vi "Configure Sweep Mode.vi"(8 "error in (no error)":errorcluster, 10 "Sweep Mode":enum16{"Continuous", "Single"}(ring), 11 "SA-ESA in":refnum<class "SA-ESA.lvclass">) -> (0 "error out":errorcluster, 3 "SA-ESA out":refnum<class "SA-ESA.lvclass">)   [LabVIEW 2020, in "SA-ESA.lvclass"]
uses:
  SA-ESA.lvclass
  C:/Sandbox/Git_Sandbox/WiSpry Test Framework source code (LV20)/WiSpry Test Framework/Instruments/Instrument.lvclass
  Instrument.lvclass/Instrument.ctl
  Instrument.lvclass
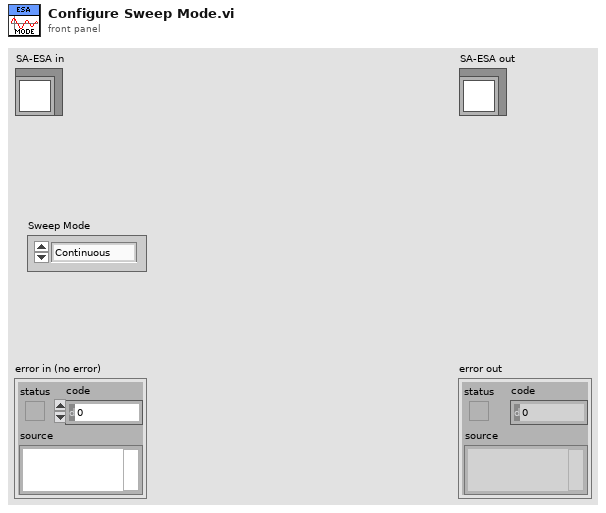
[diagram p1: front panel]
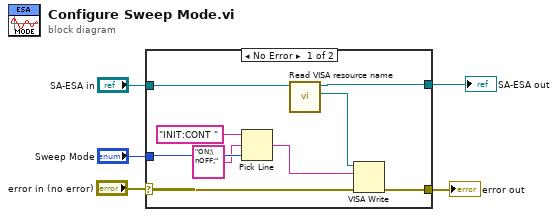
[diagram p0: block diagram]
diagram:
  n1 = case shown="No Error" "error in (no error)" {
    selector: "error in (no error)" -> [w8 w15]
    tunnel: "SA-ESA in" -> [w11 w16]
    tunnel: "Sweep Mode" -> [w14 _]
    tunnel: [w7 w15] -> w2
    tunnel: [w6 w16] -> w1
    frame No Error {
      n2 = Pick Line(string ("")="INIT:CONT ", multi-line string="ON;\nOFF;", line index=w14) -> (output string=w9:string)
      n3 = call "Read VISA resource name.vi"("Instrument in"=w11) -> ("VISA resource name"=w10:refnum<visa-resource-name>, "Instrument out"=w6:refnum<class "SA-ESA.lvclass">)  [unwired: 9 in]
      n4 = VISA Write(VISA resource name=w10, write buffer=w9, error in (no error)=w8) -> (error out=w7:errorcluster)  [unwired: 2 out]
    }
    frame Error {
    }
  }
  "error out" <- w2
  "SA-ESA out" <- w1
